vi "Write Description.vi"(8 "error in (no error)":errorcluster, 10 "Description":string, 11 "Room Service Monitor UI in":refnum<class "Room Service Monitor UI.lvclass">) -> (0 "error out":errorcluster, 3 "Room Service Monitor UI out":refnum<class "Room Service Monitor UI.lvclass">)   [LabVIEW 2023, in "Room Service Monitor UI.lvlib" / "Room Service Monitor UI.lvclass"]
uses:
  Room Service Monitor UI.lvclass
  Room Service Monitor UI.lvclass/Room Service Monitor UI.ctl
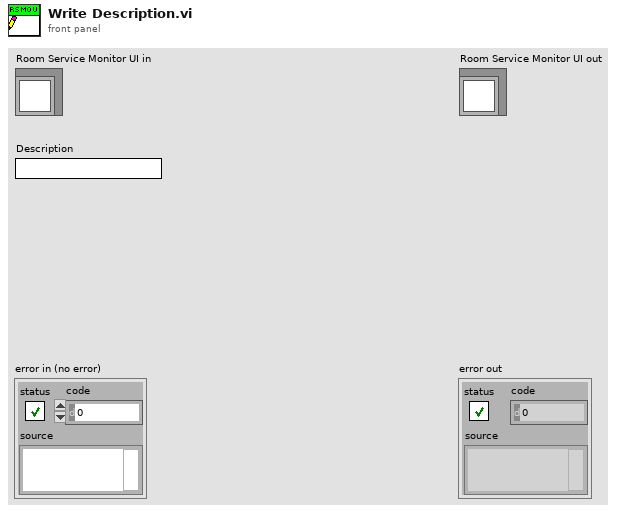
[diagram p1: front panel]
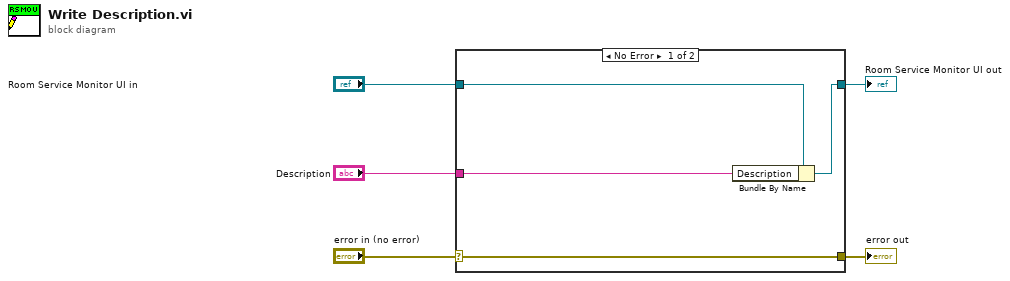
[diagram p0: block diagram]
diagram:
  n1 = case shown="No Error" "error in (no error)" {
    selector: "error in (no error)" -> [w9 w10]
    tunnel: [w9 w10] -> w4
    tunnel: [w7 w11] -> w2
    tunnel: "Room Service Monitor UI in" -> [w8 w11]
    tunnel: "Description" -> [w6 _]
    frame No Error {
      n2 = Bundle By Name(cluster=w8, "Description"=w6) -> (w7:refnum<class "Room Service Monitor UI.lvclass">)
    }
    frame Error {
    }
  }
  "error out" <- w4
  "Room Service Monitor UI out" <- w2
